vi "Pre Launch Init.vi"(11 "cRIO Vacuum in":refnum<class "cRIO Vacuum.lvclass">) -> (0 "error out":errorcluster, 3 "cRIO Vacuum out":refnum<class "cRIO Vacuum.lvclass">)   [LabVIEW 2015, in "cRIO-Carbondioxide.lvlib" / "CO2-Actor.lvlib" / "cRIO Vacuum.lvclass"]
doc: "(<B>Filename</B>: Actor Framework.lvlib:Actor.lvclass:Pre Launch Init.vi)\n\nDefines behavior that occurs after the Launch Actor method is invoked but before the actor's Actor Core method begins running.\n\nThe Pre Launch Init method is guaranteed to finish before the Launch Actor method returns to its caller and before the actor itself receives any messages. Any references that the Pre Launch Init method obtains are guaranteed to have the same lifetime as the actor itself. Any errors that the Pre Launch Init method returns will abort the launch.\n\nBy default, this method does nothing. A descendant class may override it to define behavior."
uses:
  cRIO Vacuum.lvclass
  CO2 Actor Messages/Timeout Msg/Timeout Msg.lvclass
  Controls/Vacuum State Enumerator.ctl
  cRIO Vacuum.lvclass/cRIO Vacuum.ctl
  <vilib>/ActorFramework/Actor/Actor.lvclass/Actor.ctl
  <vilib>/ActorFramework/Message Enqueuer/Message Enqueuer.lvclass/Message Enqueuer.ctl
  <vilib>/ActorFramework/Actor/Read Self Enqueuer.vi
  <vilib>/ActorFramework/Message Enqueuer/Init from Existing Queue.vi
  CO2 Actor/CO2 Actor.lvclass
  <vilib>/ActorFramework/Message Enqueuer/Message Enqueuer.lvclass
  <vilib>/ActorFramework/Actor/Actor.lvclass
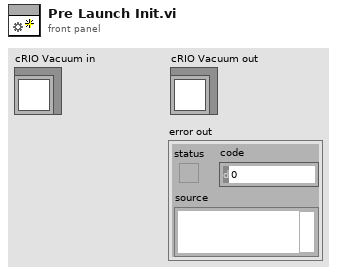
[diagram p1: front panel]
types:
  T1 = typedef "Vacuum State Enumerator.ctl" = enum16{"Pressure Rising", "Plateau", "Pressure Dropping", "Valley", "Low Valley", "Leak", "Unknown"}
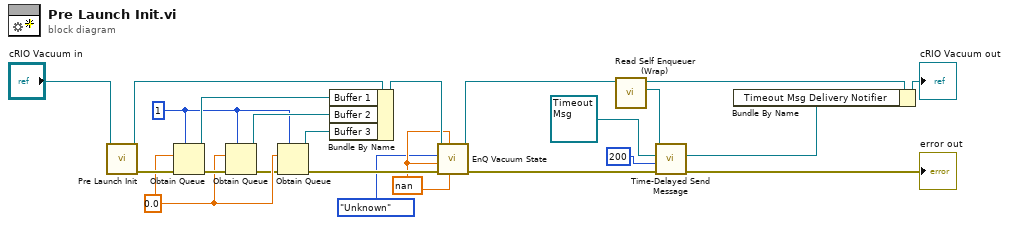
[diagram p0: block diagram]
diagram:
  w4 = nan ("Pressure")
  w9 = 0.0
  w6 = 1 ("max queue size (-1, unlimited)")
  n1 = call-parent "Pre Launch Init.vi"("CO2 Actor in"="cRIO Vacuum in") -> ("error out"=w14:errorcluster, "CO2 Actor out"=w21:refnum<class "cRIO Vacuum.lvclass">)  [unwired: 9 in]
  n2 = Obtain Queue(max queue size (-1, unlimited)=w6, element data type=w9, error in (no error)=w14) -> (queue out=w12:refnum<queue>, error out=w13:errorcluster)  [unwired: 2 in, 1 out]
  n3 = Obtain Queue(max queue size (-1, unlimited)=w6, element data type=w9, error in (no error)=w13) -> (queue out=w11:refnum<queue>, error out=w8:errorcluster)  [unwired: 2 in, 1 out]
  n4 = Obtain Queue(max queue size (-1, unlimited)=w6, element data type=w9, error in (no error)=w8) -> (queue out=w5:refnum<queue>, error out=w7:errorcluster)  [unwired: 2 in, 1 out]
  n5 = Bundle By Name(cluster=w21, "Buffer 1"=w12, "Buffer 2"=w11, "Buffer 3"=w5) -> (w10:refnum<class "cRIO Vacuum.lvclass">)
  n6 = call "EnQ Vacuum State.vi"("Raw Pressure"=w4, "d/dt"=w4, "error in (no error)"=w7, "Pressure"=w4, "State"=Vacuum_State_Enumerator."Unknown", "cRIO Vacuum in"=w10) -> ("error out"=w1:errorcluster, "cRIO Vacuum out"=w2:refnum<class "cRIO Vacuum.lvclass">)  [unwired: 4 out]
  n7 = call "Read Self Enqueuer (Wrap).vi"("CO2 Actor in"=w2) -> ("Actor Framework:Message Enqueuer"=w19:refnum<class "Message Enqueuer.lvclass">, "CO2 Actor out"=w20:refnum<class "cRIO Vacuum.lvclass">)  [unwired: 9 in]
  n8 = call <vilib>:"Time-Delayed Send Message.vi"("error in (no error)"=w1, "Milliseconds To Wait"=200, "Message"=refnum<class "Timeout Msg.lvclass"> refnum ("Timeout Msg.lvclass"), "Message Enqueuer"=w19) -> ("error out"=→"error out":errorcluster, "Delivery Notifier"=w15:refnum<notifier>)  [unwired: 6 in]
  n9 = Bundle By Name(cluster=w20, "Timeout Msg Delivery Notifier"=w15) -> (→"cRIO Vacuum out":refnum<class "cRIO Vacuum.lvclass">)
